vi "NLR4.vi"(10 "X2":dbl) -> (2 "s? t:f":dbl)   [LabVIEW 2013]
uses:
  <vilib>/express/express arith-compare/Formula/XNode/ExpressFormulaBlockNode.xnode
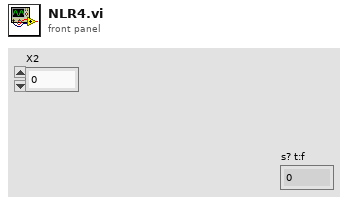
[diagram p1: front panel]
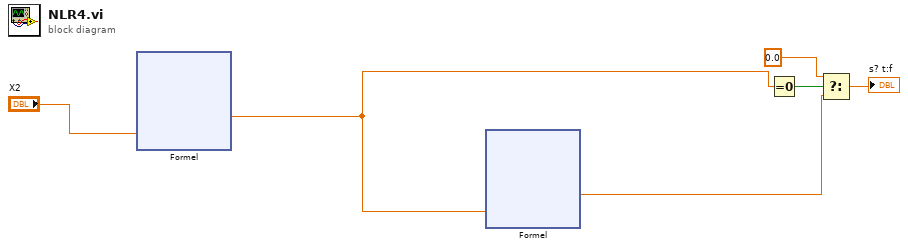
[diagram p0: block diagram]
diagram:
  n1 = xnode "Formel"("X2"="X2") -> ("Ergebnis"=w2:dbl)  [unwired: 1 in, 1 out]
  n2 = xnode "Formel"("b"=w2) -> ("Ergebnis"=w3:dbl)  [unwired: 1 in, 1 out]
  n3 = Equal To 0? ("Gleich 0?")(x=w2) -> (x = 0?=w6:bool)
  n4 = Select ("Auswählen")(t=0.0 ("value below threshold 2"), s=w6, f=w3) -> (s? t:f=→"s? t:f":dbl)
